vi "resultant_force_check.vi"(8 "reaction":dbl, 9 "drag_magnitude":dbl, 10 "propeller_horizontal_force":dbl, 11 "angle_input":i16) -> (1 "angle_out":dbl, 2 "resultant_y_force":dbl, 3 "resultant_x_force":dbl)   [LabVIEW 2018]
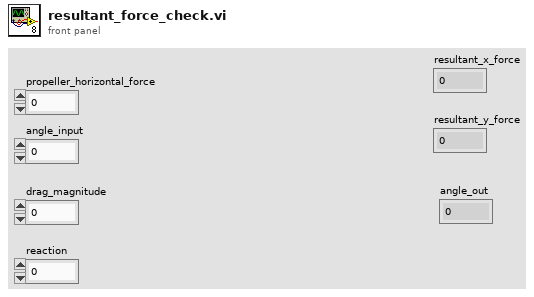
[diagram p1: front panel]
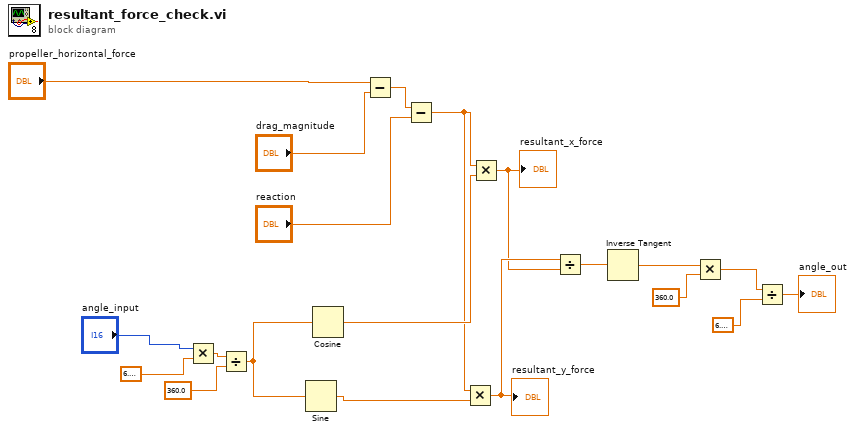
[diagram p0: block diagram]
diagram:
  n1 = Multiply(x="angle_input", y=6.283185307179586) -> (x*y=w18:dbl)
  n2 = Divide(x=w18, y=360.0) -> (x/y=w15:dbl)
  n3 = Sine(x=w15) -> (sin(x)=w9:dbl)
  n4 = Cosine(x=w15) -> (cos(x)=w11:dbl)
  n5 = Subtract(x="propeller_horizontal_force", y="drag_magnitude") -> (x-y=w20:dbl)
  n6 = Subtract(x=w20, y="reaction") -> (x-y=w10:dbl)
  n7 = Multiply(x=w10, y=w9) -> (x*y=w8:dbl)
  "resultant_y_force" <- w8
  n8 = Multiply(x=w10, y=w11) -> (x*y=w7:dbl)
  "resultant_x_force" <- w7
  n9 = Divide(x=w8, y=w7) -> (x/y=w6:dbl)
  n10 = Inverse Tangent(1:w6) -> (0:w5:dbl)
  n11 = Multiply(x=w5, y=360.0) -> (x*y=w3:dbl)
  n12 = Divide(x=w3, y=6.283185307179586) -> (x/y=→"angle_out":dbl)
